vi "sin.vi"() -> ()   [LabVIEW 2019]
panel:
  out "Array":cluster{"X":dbl, "Y":dbl}[](array[cluster])
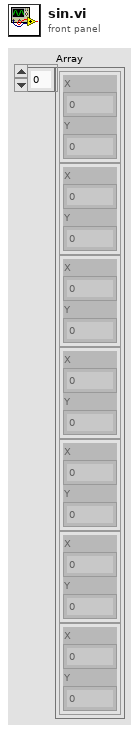
[diagram p1: front panel]
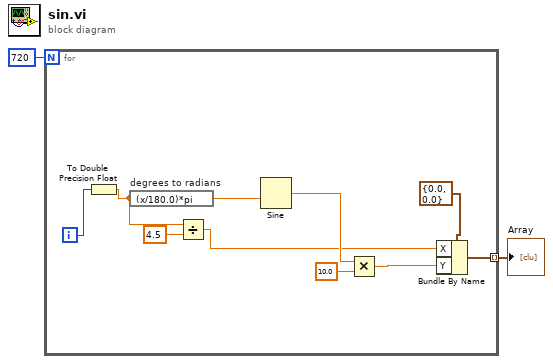
[diagram p0: block diagram]
diagram:
  n1 = for {
    N: 720 -> [_]
    tunnel: [w3] -> w1 mode=indexing
    i -> [w12]
    n2 = To Double Precision Float(number=w12) -> (double precision float=w6:dbl)
    n3 = expression code="(x/180.0)*pi" "degrees to radians"(w6) -> (w11:dbl)
    n4 = Divide(x=w6, y=4.5) -> (x/y=w4:dbl)
    n5 = Sine(x=w11) -> (sin(x)=w9:dbl)
    n6 = Multiply(x=w9, y=10.0) -> (x*y=w7:dbl)
    n7 = Bundle By Name(cluster=cluster{"X":dbl, "Y":dbl} {"X"=0.0, "Y"=0.0} ("Cluster"), "X"=w4, "Y"=w7) -> (w3:cluster{"X":dbl, "Y":dbl})
  }
  "Array" <- w1
